vi "SHAPE_readSearchType.vi"(8 "error in (no error)":errorcluster, 11 "BandGlobalOpt in":refnum<class "Shapelets Search GA.lvclass">) -> (0 "error out":errorcluster, 2 "ClassifierTypes":T1, 3 "BandGlobalOpt out":refnum<class "Shapelets Search GA.lvclass">)   [LabVIEW 2016, in "Shapelets Search (GA).lvlib" / "Shapelets Search GA.lvclass"]
uses:
  Shapelets Search GA.lvclass
  SHAPE_SearchTypes.ctl
  Shapelets Search GA.lvclass/Shapelets Search GA.ctl
  Shapelets Search (GA).lvlib
panel:
  # "This VI is a part of BCI Design library, http://www.ru-bci.org \nCopyright © 2020, Sotnikov Peter, All rights reserved. License: CC BY-NC 4.0"
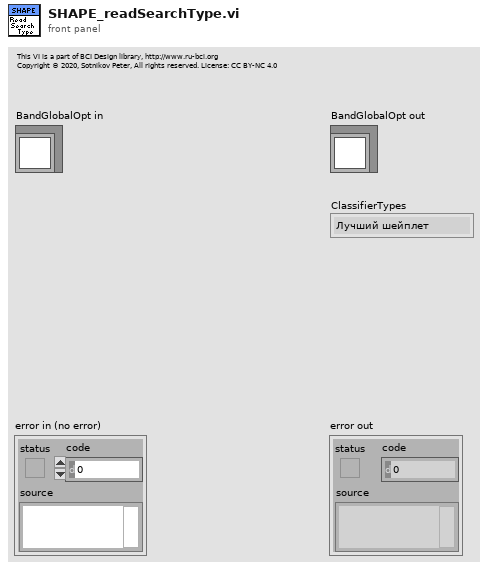
[diagram p1: front panel]
types:
  T1 = typedef "Shapelets Search (GA).lvlib/SHAPE_SearchTypes.ctl" = enum16{"Лучший шейплет", "Набор шейплетов"}
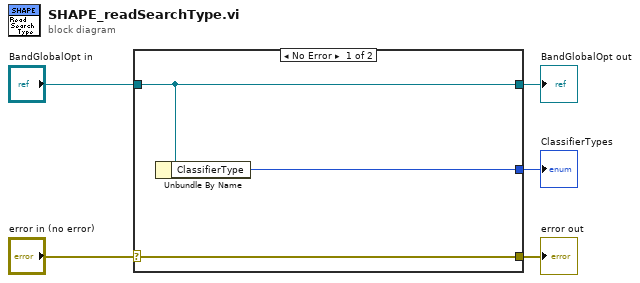
[diagram p0: block diagram]
diagram:
  n1 = case shown="No Error" "error in (no error)" {
    selector: "error in (no error)" -> [w8 w9]
    tunnel: [w8 w9] -> w4
    tunnel: [w7 w10] -> w2
    tunnel: "BandGlobalOpt in" -> [w7 w10]
    tunnel: [w6 _] -> w1
    frame No Error {
      n2 = Unbundle By Name(w7) -> ("ClassifierType"=w6:T1)
    }
    frame Error {
    }
  }
  "error out" <- w4
  "BandGlobalOpt out" <- w2
  "ClassifierTypes" <- w1
